vi "Cargo Angle Thing Controller.vi"(8 "error in":errorcluster) -> ()   [LabVIEW 2018]
doc: "This VI executes continuously carrying out the current operation and responding to updates or new operations. It will often contain the timing or control code that is difficult to place directly in TeleOp. This VI generally opens all sensors and motors and isolates the rest of the robot code from knowing how the operations are carried out."
uses:
  <vilib>/Rock Robotics/WPI/Framework/Completion Status.ctl
  Cargo Angle Thing Setpoints.ctl
  Cargo Angle Thing Operations.ctl
  <vilib>/Rock Robotics/WPI/ThirdParty/REV Robotics/SPARK MAX/Typedef/Spark MAX Control Type.ctl
  <vilib>/Rock Robotics/Network Tables/NT Read Boolean.vi
panel:
  out "Sensor Position":dbl
  in  "Interactive Values":T1
  out "Current\nCmd":string
  in  "Buttons":cluster{"Execute Cmd":bool, "Abort Cmd":bool}
  out "Command Timing":cluster{"Start Time (ms)":u32, "Iterations":i32}
  out "Status":T3
  # "Tip: It may be helpful to observe inputs and sensor values.\nYou may also want to display tuning or debugging controls."
  # "Interactive Command: You may fill in the settings for a command\nand schedule it with the Execute button. You can observe and abort\nany command while fine tuning the code for the controller."
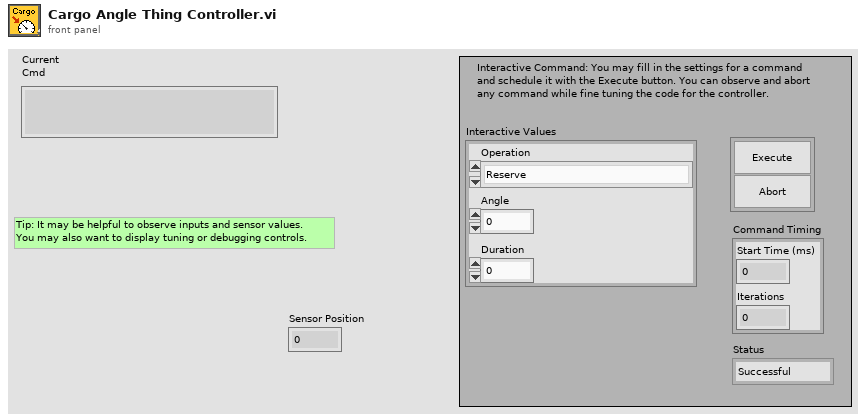
[diagram p1: front panel]
types:
  T1 = typedef "Cargo Angle Thing Setpoints.ctl" = cluster{"Operation":T2, "Angle":dbl, "Duration":dbl}
  T2 = typedef "Cargo Angle Thing Operations.ctl" = enum16{"Reserve", "Read Current", "Immediate", "Go to Position"}
  T3 = typedef "Completion Status.ctl" = enum16{"Successful", "Aborted", "Incomplete"}
  T4 = cluster{"P Gain":dbl, "I Gain":dbl, "D Gain":dbl, "F Gain":dbl, "I Zone":dbl, "Min Output":dbl, "Max Output":dbl}
  T5 = typedef "WPI_MotorControlDeviceRef.ctl" = cluster{"DeviceStatus":errorcluster, "Type":T6, "PWM":cluster{"PWM Channel":T7, "DeadBand":T8}, "CAN":cluster{"Device Number":u8, "SetOutput VI Ref":variant, "GetOutput VI Ref":variant, "Enable VI Ref":variant, "Disable VI Ref":variant, "Data":variant}, "Invert":bool, "DIO PWM":cluster{"PWM \"Enable\" Channel":T7, "DIOChannel":T9, "PWM Rate":dbl}}
  T6 = typedef "WPI_MotorControlType.ctl" = enum16{"PWM", "CAN", "DIO PWM"}
  T7 = typedef "FPGA_DIOPWMChannel.ctl" = enum8{"PWM 0", "PWM 1", "PWM 2", "PWM 3", "PWM 4", "PWM 5", "PWM 6", "PWM 7", "PWM 8", "PWM 9", "PWM MXP 0", "PWM MXP 1", "PWM MXP 2", "PWM MXP 3", "PWM MXP 4", "PWM MXP 5", "PWM MXP 6", "PWM MXP 7", "PWM MXP 8", "PWM MXP 9", "Invalid"}
  T8 = typedef "WPI_PWMDeadband.ctl" = cluster{"Name":string, "maxPositivePwm":i32, "minPositivePwm":i32, "centerPwm":i32, "maxNegativePwm":i32, "minNegativePwm":i32, "angularRange":u16}
  T9 = typedef "FPGA_DIOChannel.ctl" = enum8{"DIO 0", "DIO 1", "DIO 2", "DIO 3", "DIO 4", "DIO 5", "DIO 6", "DIO 7", "DIO 8", "DIO 9", "DIO MXP 0", "DIO MXP 1", "DIO MXP 2", "DIO MXP 3", "DIO MXP 4", "DIO MXP 5", "DIO MXP 6", "DIO MXP 7", "DIO MXP 8", "DIO MXP 9", "DIO MXP 10", "DIO MXP 11", "DIO MXP 12", "DIO MXP 13", "DIO MXP 14", "DIO MXP 15", "SPI Port CS1", "SPI Port CS2", "SPI Port CS3", "SPI Port MISO", "SPI Port MOSI", "Invalid"}
  T10 = typedef "Command Status Info.ctl" = cluster{"Name":string, "Status":T3, "notifier out":T11}
  T11 = typedef "Completion Notifier.ctl" = refnum<notifier>
  T12 = cluster{"Current Command":T1, "Command Timing":cluster{"Start Time (ms)":u32, "Iterations":i32}, "Command Arguments":cluster{"Command Info":T10, "Description":string, "Default Command":T1, "queue out":refnum<queue>, "Subsystem Name":string}}
  T13 = typedef "Spark MAX Control Type.ctl" = enum16{"Percent VBus", "Voltage", "Velocity", "Position", "Smart Motion", "Current", "Smart Velocity"}
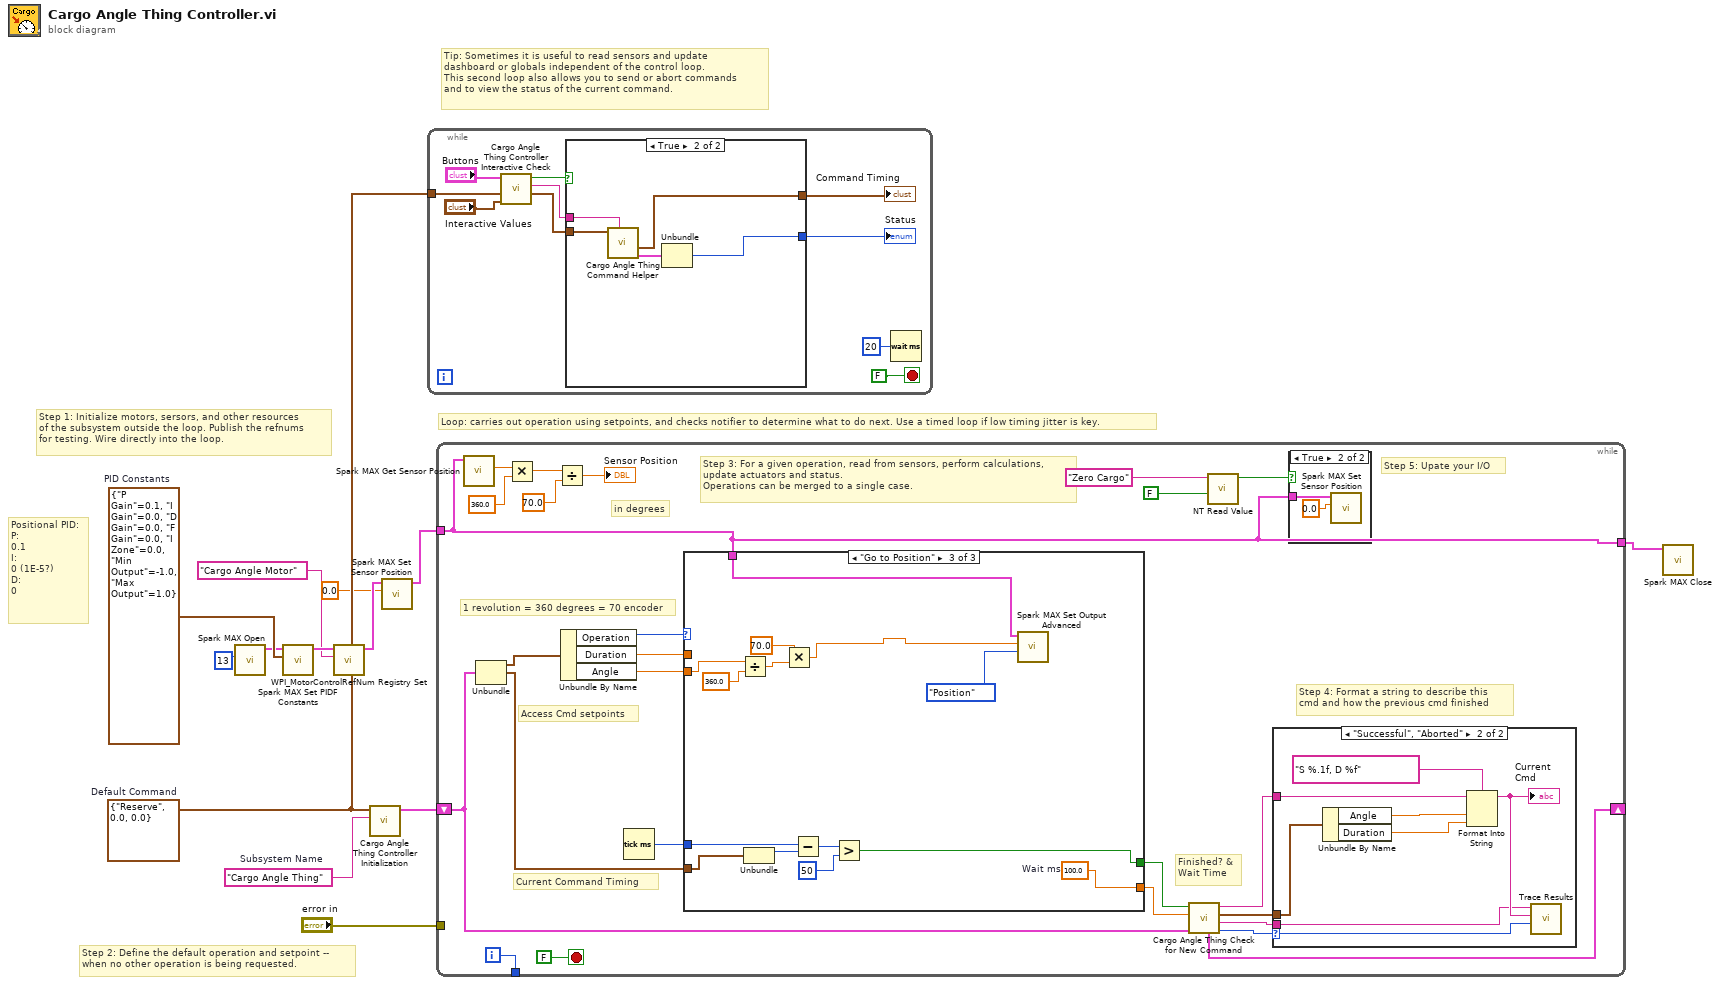
[diagram p0: block diagram]
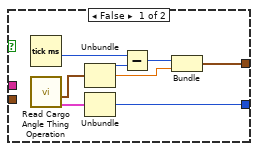
[diagram p2: hidden frame]
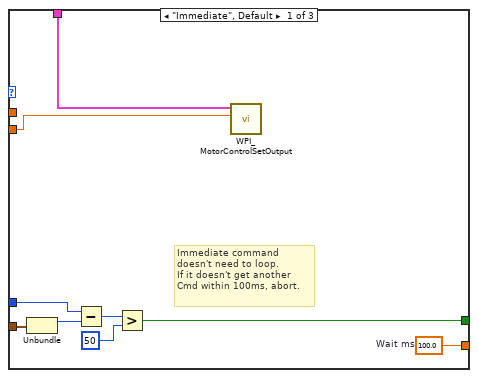
[diagram p5: hidden frame]
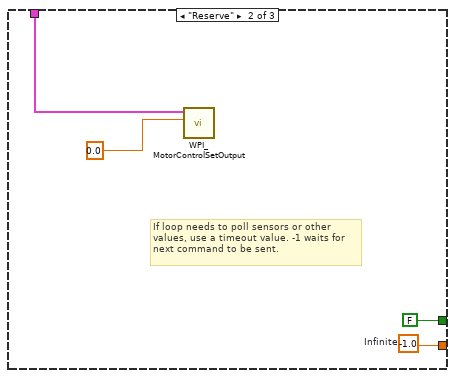
[diagram p6: hidden frame]
diagram:
  w8 = T4 {"P Gain"=0.1, "I Gain"=0.0, "D Gain"=0.0, "F Gain"=0.0, "I Zone"=0.0, "Min Output"=-1.0, "Max Output"=1.0}  # PID Constants
  w10 = T1 {"Operation"=enum."Reserve", "Angle"=0.0, "Duration"=0.0}  # Default Command
  w11 = "Cargo Angle Thing"  # Subsystem Name
  # "Positional PID:\nP:\n0.1\nI:\n0 (1E-5?)\nD:\n0"
  # "Tip: Sometimes it is useful to read sensors and update\ndashboard or globals independent of the control loop.\nThis second loop also allows you to send or abort commands\nand to view the status of the current command."
  # "Step 2: Define the default operation and setpoint --\nwhen no other operation is being requested."
  # "Step 1: Initialize motors, sersors, and other resources\nof the subsystem outside the loop. Publish the refnums\nfor testing. Wire directly into the loop."
  # "Loop: carries out operation using setpoints, and checks notifier to determine what to do next. Use a timed loop if low timing jitter is key."
  n1 = call <vilib>:"Spark MAX Open.vi"("Device Number"=u8 13) -> ("MotorControlDeviceRef"=w7:T5)  [unwired: 9 in, 1 out]
  n2 = call <vilib>:"Spark MAX Set PIDF Constants.vi"("PID Constants"=w8, "MotorControlDeviceRef"=w7) -> ("MotorControlDeviceRef"=w4:T5)  [unwired: 8 in, 1 out]
  n3 = call <vilib>:"WPI_MotorControlRefNum Registry Set.vi"("refnum name"="Cargo Angle Motor", "MotorControlDevRef"=w4) -> ("MotorControlDevRef"=w3:T5)  [unwired: 8 in, 1 out]
  n4 = call "Cargo Angle Thing Controller Initialization.vi"("Subsystem Name"=w11, "Default Command"=w10) -> ("Current Command"=w12:T12)  [unwired: 9 in]
  n5 = call <vilib>:"Spark MAX Set Sensor Position.vi"("Position"=0.0, "MotorControlDeviceRef"=w3) -> ("MotorControlDeviceRef"=w6:T5)  [unwired: 8 in, 1 out]
  n6 = while {
    tunnel: w10 -> [w20]
    stop <- FALSE stop-if-true
    n7 = call "Cargo Angle Thing Controller Interactive Check.vi"("Interactive Command in"="Interactive Values", "Default Command"=w20, "Buttons"="Buttons") -> ("Interactive Command out"=w17:T1, "Trace String"=w18:string, "Schedule"=w19:bool)  [unwired: 6 in]
    n8 = case shown="True" w19 {
      tunnel: [w31 w36] -> w16
      tunnel: w17 -> [_ w34]
      tunnel: [w27 w32] -> w15
      tunnel: w18 -> [_ w35]
      frame False {
        n9 = Tick Count (ms)() -> (millisecond timer value=w26:u32)
        n10 = call "Read Cargo Angle Thing Operation.vi"() -> ("Command Info"=w24:T10, "SubSystem Data"=w25:T1)  [unwired: 9 in, 1 out]
        n11 = Unbundle(w25) -> ("Operation"=w30:T2, "Angle"=w28:dbl)  [unwired: 1 out]
        n12 = Unbundle(w24) -> ("Status"=w31:T3)  [unwired: 2 out]
        n13 = Subtract(x=w26, y=w30) -> (x-y=w29:u32)
        n14 = Bundle(w29, "Angle"=w28) -> (w27:cluster{u32, "Angle":dbl})  [unwired: 1 in]
      }
      frame True {
        n15 = call "Cargo Angle Thing Command Helper.vi"("Description"=w35, "SubSystem Data"=w34) -> ("Command Info Out"=w33:T10, "Command Timing"=w32:cluster{"Start Time (ms)":u32, "Iterations":i32})  [unwired: 7 in, 1 out]
        n16 = Unbundle(w33) -> ("Status"=w36:T3)  [unwired: 2 out]
      }
    }
    "Status" <- w16
    "Command Timing" <- w15
    n17 = Wait (ms)(milliseconds to wait=u32 20) -> ()  [unwired: 1 out]
  }
  n18 = while {
    shift-right: [w54] -> _
    shift-left: w12 -> [w47]
    tunnel: [w60] -> _
    tunnel: "error in" -> [_]
    tunnel: w6 -> [w37]
    tunnel: [w37] -> w5
    i -> [w60]
    stop <- FALSE stop-if-true
    # "in degrees"
    # "1 revolution = 360 degrees = 70 encoder"
    # "Step 5: Upate your I/O"
    # "Step 4: Format a string to describe this\ncmd and how the previous cmd finished"
    # "Current Command Timing"
    # "Access Cmd setpoints"
    # "Finished? &\nWait Time"
    # "Step 3: For a given operation, read from sensors, perform calculations,\nupdate actuators and status.\nOperations can be merged to a single case."
    n19 = call <vilib>:"Spark MAX Get Sensor Position.vi"("MotorControlDevRef in"=w37) -> ("Sensor Position"=w45:dbl)  [unwired: 7 in, 3 out]
    n20 = Unbundle(w47) -> ("Current Command"=w59:T1, "Command Timing"=w56:cluster{"Start Time (ms)":u32, "Iterations":i32})  [unwired: 1 out]
    n21 = Multiply(x=w45, y=360.0) -> (x*y=w43:dbl)
    n22 = Divide(x=w43, y=70.0) -> (x/y=→"Sensor Position":dbl)
    n23 = Unbundle By Name(w59) -> ("Operation"=w58:T2, "Duration"=w57:dbl, "Angle"=w55:dbl)
    n24 = Tick Count (ms)() -> (millisecond timer value=w46:u32)
    n25 = case shown="\"Go to Position\"" w58 {
      tunnel: [w80 w84 w93] -> w52
      tunnel: [w74 FALSE ("ignore previous (F)") w92] -> w53
      tunnel: w56 -> [w76 _ w94]
      tunnel: w57 -> [_ _ _]
      tunnel: w46 -> [w75 _ w95]
      tunnel: w55 -> [w72 _ w91]
      tunnel: w37 -> [w73 w82 w87]
      frame "Immediate", Default {
        w80 = 100.0  # Wait ms
        # "Immediate command\ndoesn't need to loop.\nIf it doesn't get another\nCmd within 100ms, abort."
        n26 = Unbundle(w76) -> ("Start Time (ms)"=w79:u32)  [unwired: 1 out]
        n27 = Subtract(x=w75, y=w79) -> (x-y=w78:u32)
        n28 = Greater?(x=w78, y=u8 50 ("Left Motor")) -> (0:w74:bool)
        n29 = call <vilib>:"WPI_MotorControlSetOutput.vi"("Output"=w72, "MotorControlDevRef"=w73) -> ()  [unwired: 7 in, 3 out]
      }
      frame "Reserve" {
        w84 = -1.0  # Infinite
        # "If loop needs to poll sensors or other\nvalues, use a timeout value. -1 waits for\nnext command to be sent."
        n30 = call <vilib>:"WPI_MotorControlSetOutput.vi"("Output"=0.0, "MotorControlDevRef"=w82) -> ()  [unwired: 7 in, 3 out]
      }
      frame "Go to Position" {
        w93 = 100.0  # Wait ms
        n31 = Divide(x=w91, y=360.0) -> (x/y=w89:dbl)
        n32 = Unbundle(w94) -> ("Start Time (ms)"=w98:u32)  [unwired: 1 out]
        n33 = Multiply(x=70.0, y=w89) -> (x*y=w85:dbl)
        n34 = Subtract(x=w95, y=w98) -> (x-y=w97:u32)
        n35 = Greater?(x=w97, y=u8 50 ("Left Motor")) -> (0:w92:bool)
        n36 = call <vilib>:"Spark MAX Set Output Advanced.vi"("Control Mode"=Spark_MAX_Control_Type."Position", "Setpoint"=w85, "MotorControlDevRef"=w87) -> ()  [unwired: 7 in, 2 out]
      }
    }
    n37 = call "Cargo Angle Thing Check for New Command.vi"("Current Command"=w47, "Wait time (ms)"=w52, "Finished?"=w53) -> ("Completion"=w48:T3, "Subsystem Name"=w49:string, "Current Command"=w50:T1, "Initial Trace String"=w51:string, "NextCommand"=w54:T12)  [unwired: 4 in]
    n38 = call-poly <vilib>:"NT Read Value.vi"("Default Value"=FALSE, "Name"="Zero Cargo") -> ("Boolean"=w38:bool)  [unwired: 8 in, 1 out]
    n39 = case shown="\"Successful\", \"Aborted\"" w48 {
      selector: w48 -> [_ w71]
      tunnel: w51 -> [_ w67]
      tunnel: w50 -> [_ w68]
      tunnel: w49 -> [_ w64]
      frame "Incomplete", Default {
        # "Continuing current command"
      }
      frame "Successful", "Aborted" {
        # "Report and setup for next command"
        n40 = Unbundle By Name(w68) -> ("Angle"=w70:dbl, "Duration"=w65:dbl)
        n41 = Format Into String(format string="S %.1f, D %f", initial string=w67, w70, w65) -> (resulting string=w66:string)  [unwired: 1 in, 1 out]
        "Current\nCmd" <- w66
        n42 = call <vilib>:"Trace Results.vi"("Status of previous command"=w71, "Description"=w66, "Subsystem"=w64) -> ()  [unwired: 9 in]
      }
    }
    n43 = case shown="True" w38 {
      tunnel: w37 -> [_ w62]
      frame False {
      }
      frame True {
        n44 = call <vilib>:"Spark MAX Set Sensor Position.vi"("Position"=0.0, "MotorControlDeviceRef"=w62) -> ()  [unwired: 8 in, 2 out]
      }
    }
  }
  n45 = call <vilib>:"Spark MAX Close.vi"("MotorControlDeviceRef"=w5) -> ()  [unwired: 10 in, 1 out]
